vi "Generate Ramp and Flyback.vi"(5 "Raster Scan Direction":T1, 6 "FOV Center (V)":dbl, 7 "Galvo Step Size Voltages (px/V)":dbl, 9 "Px Dim (HFOV)":u16, 10 "Pixel Dwell Time [Clock Cycles]":u16, 11 "Flyback Time [Clock Cycles]":u16) -> (1 "Flyback":dbl[][](array[numeric]), 2 "Clocks Cycle":i32, 3 "Waveform Graph":dbl[](graph))   [LabVIEW 2018]
uses:
  Controls/Scan Direction.ctl
  <vilib>/Analysis/1siggen.llb/Ramp Pattern by Delta.vi
  <vilib>/Analysis/NI_AALBase.lvlib
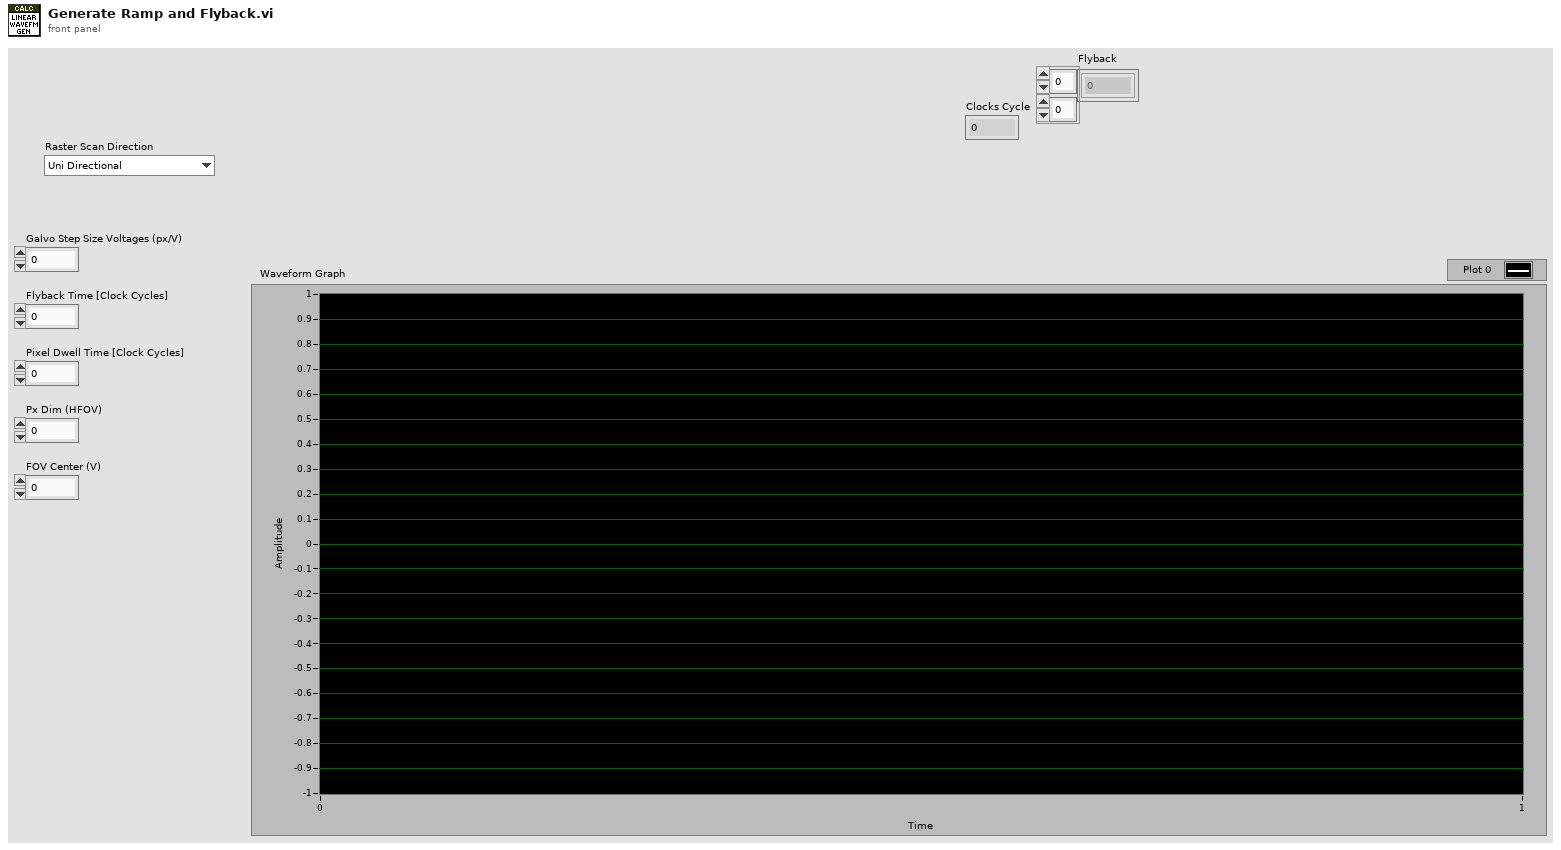
[diagram p1: front panel]
types:
  T1 = typedef "Scan Direction.ctl" = enum16{"Uni Directional", "Bi Directional", "None"}
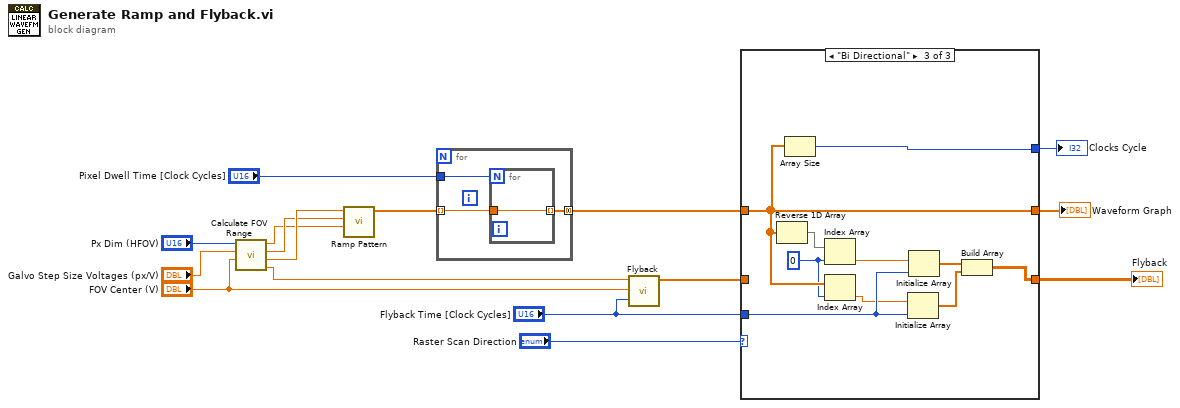
[diagram p0: block diagram]
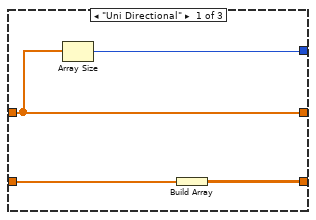
[diagram p2: hidden frame]
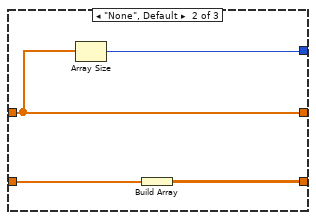
[diagram p3: hidden frame]
diagram:
  n1 = call "Calculate FOV Range.vi"("Center Voltage"="FOV Center (V)", "Galvo Step Stize (px/V)"="Galvo Step Size Voltages (px/V)", "Num. Px(Half FOV)"="Px Dim (HFOV)") -> ("Amplitude"=w9:dbl, "Galvo Step Stize (px/V) Out"=w15:dbl, "Stop Value"=w14:dbl, "Start Value"=w13:dbl)  [unwired: 5 in]
  n2 = call-poly <vilib>:"Ramp Pattern.vi"("start"=w13, "end"=w14, "delta"=w15) -> ("Ramp Pattern"=w6:dbl[])  [unwired: 6 in, 2 out]
  n3 = for {
    tunnel: w6 -> [w19] mode=indexing
    tunnel: "Pixel Dwell Time [Clock Cycles]" -> [w18]
    tunnel: [w17] -> w5 mode=concatenating
    n4 = for {
      N: w18 -> [_]
      tunnel: w19 -> [w20]
      tunnel: [w20] -> w17 mode=indexing
    }
  }
  n5 = call "Flyback.vi"("Flyback Time [Clock Cycles]"="Flyback Time [Clock Cycles]", "Center (V)"="FOV Center (V)", "Amplitude (V)"=w9) -> ("Waveform + Flyback"=w2:dbl[])  [unwired: 8 in]
  n6 = case shown="\"Bi Directional\"" "Raster Scan Direction" {
    tunnel: "Flyback Time [Clock Cycles]" -> [_ _ w35]
    tunnel: [w21 w27 w37] -> w7
    tunnel: w5 -> [w21 w27 w37]
    tunnel: [w24 w28 w38] -> w3
    tunnel: w2 -> [w23 w26 _]
    tunnel: [w22 w25 w29] -> w1
    frame "Uni Directional" {
      n7 = Array Size(array=w21) -> (size(s)=w24:i32)
      n8 = Build Array(w23) -> (w22:dbl[][])
    }
    frame "None", Default {
      n9 = Array Size(array=w27) -> (size(s)=w28:i32)
      n10 = Build Array(w26) -> (w25:dbl[][])
    }
    frame "Bi Directional" {
      w32 = 0 ("index")
      n11 = Reverse 1D Array(array=w37) -> (reversed array=w36:dbl[])
      n12 = Array Size(array=w37) -> (size(s)=w38:i32)
      n13 = Index Array(array=w36, index=w32) -> (element=w34:dbl)
      n14 = Index Array(array=w37, index=w32) -> (element=w33:dbl)
      n15 = Initialize Array(w33, w35) -> (w30:dbl[])
      n16 = Initialize Array(w34, w35) -> (w31:dbl[])
      n17 = Build Array(w31, w30) -> (w29:dbl[][])
    }
  }
  "Waveform Graph" <- w7
  "Clocks Cycle" <- w3
  "Flyback" <- w1
